vi "Untitled 1 (SubVI).vi"(1 "reference":refnum<vi>) -> (0 "Event Registration Refnum":refnum<event-registration>)   [LabVIEW 2015, in "AguaClara Library.lvlib"]
uses:
  AguaClara Library.lvlib
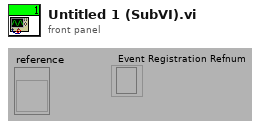
[diagram p1: front panel]
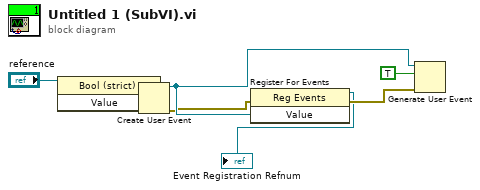
[diagram p0: block diagram]
diagram:
  n1 = property class="Bool (strict)"(reference="reference") -> ("Value"=w2:bool)  [unwired: 1 in, 2 out]
  n2 = Create User Event(user event datatype=w2) -> (user event=w7:refnum<user-event>, error out=w6:errorcluster)  [unwired: 1 in]
  n3 = register-events(error in=w6, w7) -> (reference out=→"Event Registration Refnum":refnum<event-registration>, error out=w5:errorcluster)  [unwired: 1 in]
  n4 = Generate User Event(user event=w7, event data cluster=TRUE ("event data"), error in=w5) -> ()  [unwired: 1 in, 2 out]
